vi "Organise_String_Array.vi"(1 "Input Array":string[](array[string])) -> (0 "Output Array":string[](array[string]))   [LabVIEW 2016]
panel:
  out "Move Up 2":bool
  in  "OK":bool
  in  "Delete":bool
  in  "Move Down":bool
  in  "Move Up":bool
  in  "Listbox":i32[](listbox)
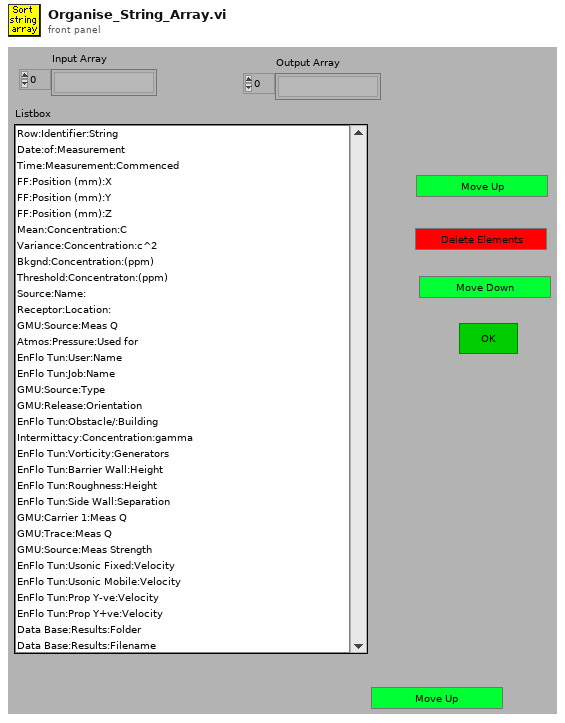
[diagram p1: front panel]
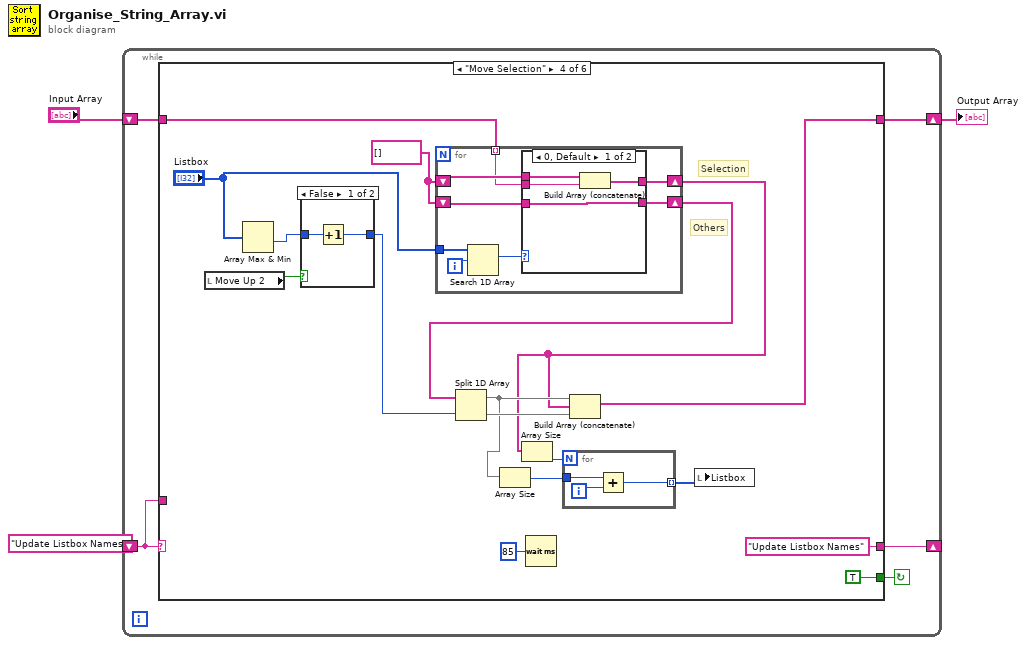
[diagram p0: block diagram]
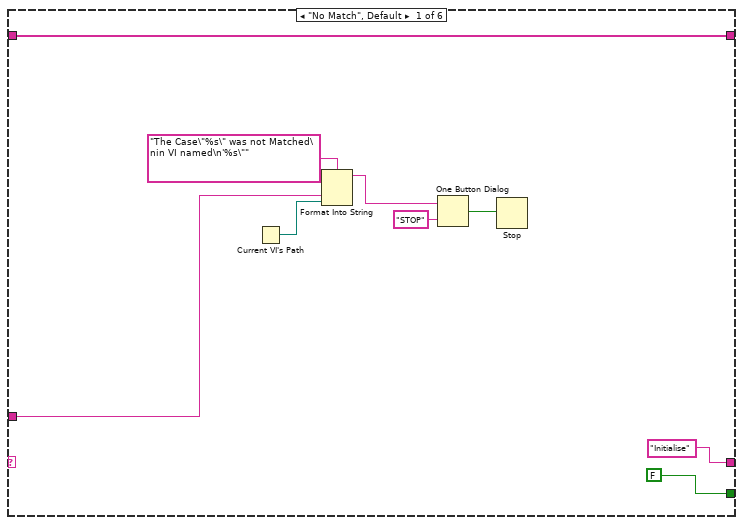
[diagram p2: hidden frame]
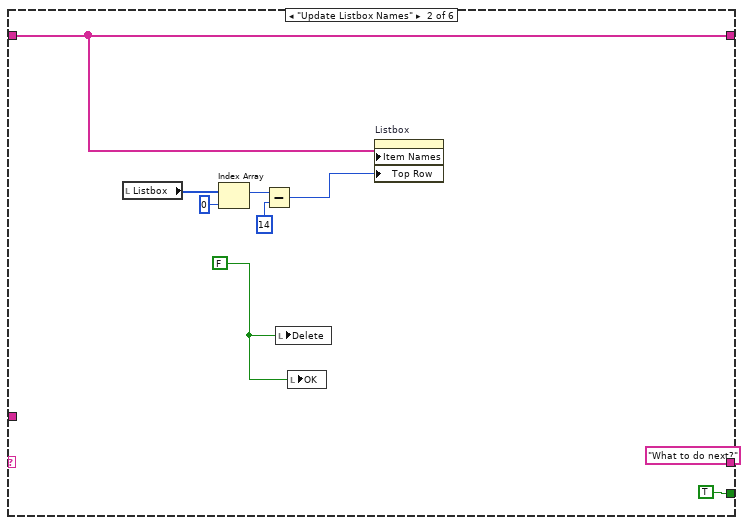
[diagram p3: hidden frame]
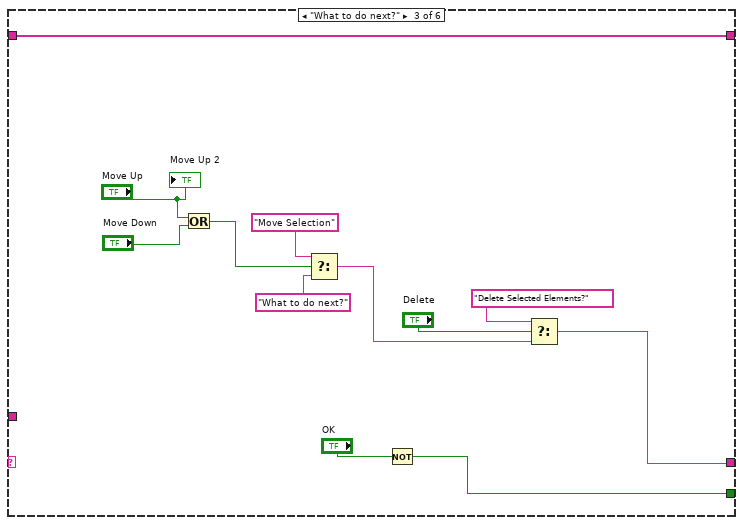
[diagram p4: hidden frame]
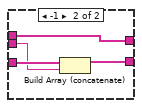
[diagram p5: hidden frame]
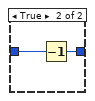
[diagram p6: hidden frame]
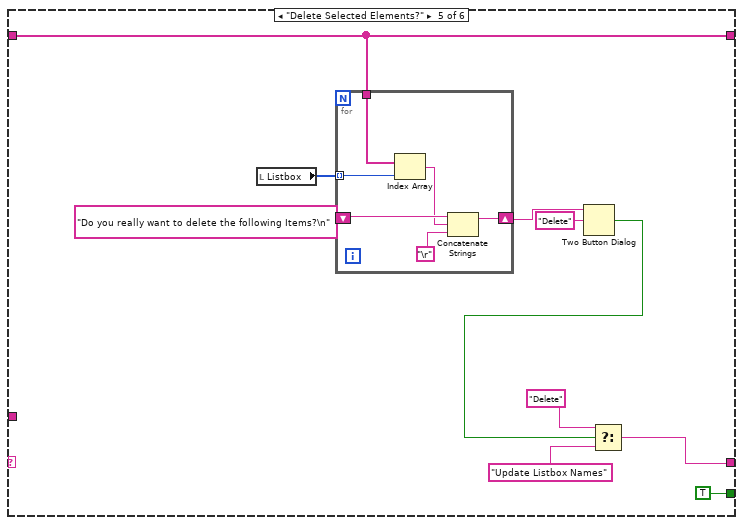
[diagram p7: hidden frame]
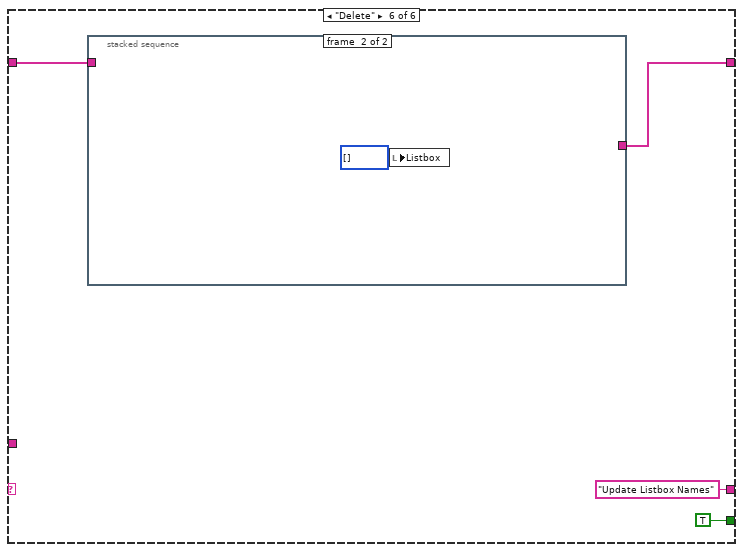
[diagram p8: hidden frame]
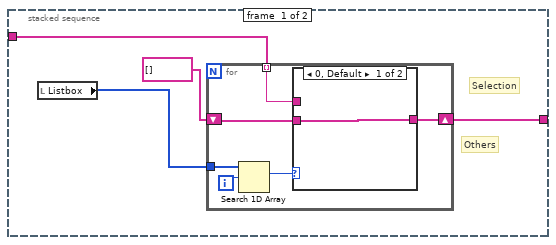
[diagram p9: hidden frame]
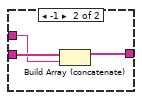
[diagram p10: hidden frame]
diagram:
  n1 = while {
    shift-left: "Input Array" -> [w5]
    shift-right: [w4] -> w1
    shift-left: "Update Listbox Names" -> [w6]
    shift-right: [w7] -> _
    stop <- w8 continue-if-true
    n2 = case shown="\"Move Selection\"" w6 {
      tunnel: [FALSE TRUE w36 TRUE TRUE TRUE] -> w8
      tunnel: ["Initialise" "What to do next?" w28 "Update Listbox Names" w80 "Update Listbox Names"] -> w7
      tunnel: w6 -> [w12 _ _ _ _ _]
      tunnel: w5 -> [w9 w24 w38 w49 w86 w98]
      tunnel: [w9 w24 w38 w48 w86 w95] -> w4
      frame "No Match", Default {
        n3 = Current VI's Path() -> (path=w11:path)
        n4 = Format Into String(format string="The Case\"%s\" was not Matched\nin VI named\n'%s\"" ("Format String"), w12, w11) -> (resulting string=w15:string)  [unwired: 2 in, 1 out]
        n5 = One Button Dialog(message=w15, button name ("OK")="STOP") -> (true=w13:bool)
        n6 = Stop(stop? (T)=w13) -> ()
      }
      frame "Update Listbox Names" {
        w23 = FALSE
        n7 = local read "Listbox"() -> (w19:i32[])
        n8 = Index Array(array=w19, index=0 ("Index")) -> (element=w21:i32)
        n9 = Subtract(x=w21, y=14) -> (x-y=w18:i32)
        n10 = local write "Delete"(w23) -> ()
        n11 = local write "OK"(w23) -> ()
        n12 = property on="Listbox" class="LstBox (strict)"("Item Names"=w24, "Top Row"=w18) -> ()  [unwired: 2 in, 2 out]
      }
      frame "What to do next?" {
        n13 = Or(x="Move Up", y="Move Down") -> (x .or. y?=w32:bool)
        n14 = Select(t="Move Selection", s=w32, f="What to do next?") -> (s? t:f=w30:string)
        n15 = Not(x="OK") -> (.not. x?=w36:bool)
        n16 = Select(t="Delete Selected Elements?", s="Delete", f=w30) -> (s? t:f=w28:string)
        "Move Up 2" <- "Move Up"
      }
      frame "Move Selection" {
        w54 = string[] []
        # "Others"
        # "Selection"
        n17 = local read "Move Up 2"() -> (w55:bool)
        n18 = Array Max & Min(array="Listbox") -> (min value=w50:i32)  [unwired: 3 out]
        n19 = case shown="False" w55 {
          tunnel: w50 -> [w76 w78]
          tunnel: [w75 w77] -> w47
          frame False {
            n20 = Increment(x=w76) -> (x+1=w75:i32)
          }
          frame True {
            n21 = Decrement(x=w78) -> (x-1=w77:i32)
          }
        }
        n22 = for {
          tunnel: "Listbox" -> [w65]
          shift-right: [w61] -> w44
          shift-left: w54 -> [w63]
          shift-right: [w59] -> w53
          shift-left: w54 -> [w60]
          tunnel: w49 -> [w62] mode=indexing
          i -> [w66]
          n23 = Search 1D Array(1D array=w65, element=w66) -> (index of element=w64:i32)  [unwired: 1 out]
          n24 = case shown="0, Default" w64 {
            tunnel: w63 -> [w70 w72]
            tunnel: w62 -> [w69 w73]
            tunnel: [w68 w72] -> w61
            tunnel: w60 -> [w67 w74]
            tunnel: [w67 w71] -> w59
            frame 0, Default {
              n25 = Build Array (concatenate)(w70, w69) -> (w68:string[])
            }
            frame -1 {
              n26 = Build Array (concatenate)(w74, w73) -> (w71:string[])
            }
          }
        }
        n27 = Split 1D Array(array=w53, index=w47) -> (first subarray=w46:string[], second subarray=w52:string[])
        n28 = Array Size(array=w46) -> (size(s)=w45:i32)
        n29 = Array Size(array=w44) -> (size(s)=w43:i32)
        n30 = Wait (ms)(milliseconds to wait=u32 85) -> ()  [unwired: 1 out]
        n31 = for {
          N: w43 -> [_]
          tunnel: w45 -> [w57]
          tunnel: [w56] -> w40 mode=indexing
          i -> [w58]
          n32 = Add(x=w57, y=w58) -> (x+y=w56:i32)
        }
        n33 = Build Array (concatenate)(w46, w44, w52) -> (w48:string[])
        n34 = local write "Listbox"(w40) -> ()
      }
      frame "Delete Selected Elements?" {
        n35 = local read "Listbox"() -> (w87:i32[])
        n36 = for {
          tunnel: w87 -> [w94] mode=indexing
          tunnel: w86 -> [w93]
          shift-right: [w89] -> w84
          shift-left: "Do you really want to delete the following Items?\n" -> [w92]
          n37 = Index Array(array=w93, index=w94) -> (element=w90:string)
          n38 = Concatenate Strings(w92, w90, "\r") -> (w89:string)
        }
        n39 = Two Button Dialog(message=w84, 2:"Delete" ("T button name (\"OK\")")) -> (T button?=w83:bool)  [unwired: 1 out]
        n40 = Select(t="Delete", s=w83, f="Update Listbox Names") -> (s? t:f=w80:string)
      }
      frame "Delete" {
        n41 = stacked-sequence {
          tunnel: w98 -> [w101 _]
          tunnel: [w99 _] -> w95
          frame #0 {
            # "Others"
            # "Selection"
            n42 = local read "Listbox"() -> (w100:i32[])
            n43 = for {
              tunnel: w100 -> [w107]
              shift-right: [w103] -> w99
              shift-left: string[] [] -> [w104]
              tunnel: w101 -> [w105] mode=indexing
              i -> [w108]
              n44 = Search 1D Array(1D array=w107, element=w108) -> (index of element=w106:i32)  [unwired: 1 out]
              n45 = case shown="0, Default" w106 {
                tunnel: w105 -> [_ w111]
                tunnel: w104 -> [w109 w112]
                tunnel: [w109 w110] -> w103
                frame 0, Default {
                }
                frame -1 {
                  n46 = Build Array (concatenate)(w112, w111) -> (w110:string[])
                }
              }
            }
          }
          frame #1 {
            n47 = local write "Listbox"(i32[] [] ("Listbox")) -> ()
          }
        }
      }
    }
  }
  "Output Array" <- w1
